vi "element_editor_save.vi"(10 "Specification Path":refnum<vi>, 11 "Parameters Tree":refnum<vi>) -> ()   [LabVIEW 2019]
uses:
  lib/libSpecValiReader/libSpecValiReader.lvlib
panel:
  # "*******************************************************************\nBiogas Plant Control\n\nAuthor: Paul Zügel\nGCSC-Frankfurt am Main 2020\n\n*******************************************************************"
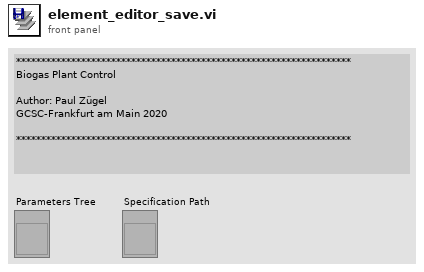
[diagram p1: front panel]
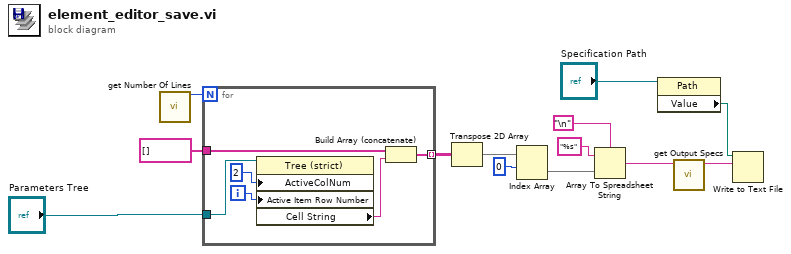
[diagram p0: block diagram]
diagram:
  n1 = call "get Number Of Lines.vi"() -> ("function return"=w4:i32)  [unwired: 10 in, 1 out]
  n2 = for {
    N: w4 -> [_]
    tunnel: string[] [] ("Empty Val Arr") -> [w17]
    tunnel: [w16] -> w11 mode=indexing
    tunnel: "Parameters Tree" -> [w14]
    i -> [w19]
    n3 = property on="Property Node" class="Tree (strict)"(reference=w14, "ActiveColNum"=2 ("Active Cell:Active Column Number"), "Active Item Row Number"=w19) -> ("Cell String"=w15:string)  [unwired: 1 in, 2 out]
    n4 = Build Array (concatenate)(w17, w15) -> (w16:string[])
  }
  n5 = Transpose 2D Array(2D array=w11) -> (transposed array=w10:string[][])
  n6 = Index Array(array=w10, index (row)=0) -> (element=w9:string[])  [unwired: 1 in]
  n7 = Array To Spreadsheet String(delimiter (Tab)="\n", array=w9, 3:"%s" ("format string")) -> (spreadsheet string=w5:string)
  n8 = property class="Path"(reference="Specification Path") -> ("Value"=w2:path)  [unwired: 1 in, 2 out]
  n9 = call "get Output Specs.vi"("specs"=w5) -> ("output"=w1:string)  [unwired: 9 in, 1 out]
  n10 = Write to Text File(file (use dialog)=w2, text=w1) -> ()  [unwired: 2 in, 3 out]
